vi "BooleanCtlTest.vi"() -> ()   [LabVIEW 2016]
uses:
  main/apis/Setup/GetVI/GetVIByPath.vi
  main/apis/Stimulus/ValueSignal/ValueSignalByPathString.vi
  main/apis/Assert/AssertControlValue/Equal.vi
  main/Drona.lvlib
  main/apis/Setup/GetVI/GetVI.lvlib
  <vilib>/addons/_JKI Toolkits/Caraya/classes/Test/Test.lvclass
  main/apis/Stimulus/ValueSignal/ValueSignal.lvlib
  main/apis/Assert/AssertControlValue/AssertControlValue.lvlib
panel:
  out "error out":errorcluster
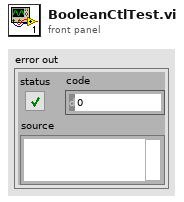
[diagram p1: front panel]
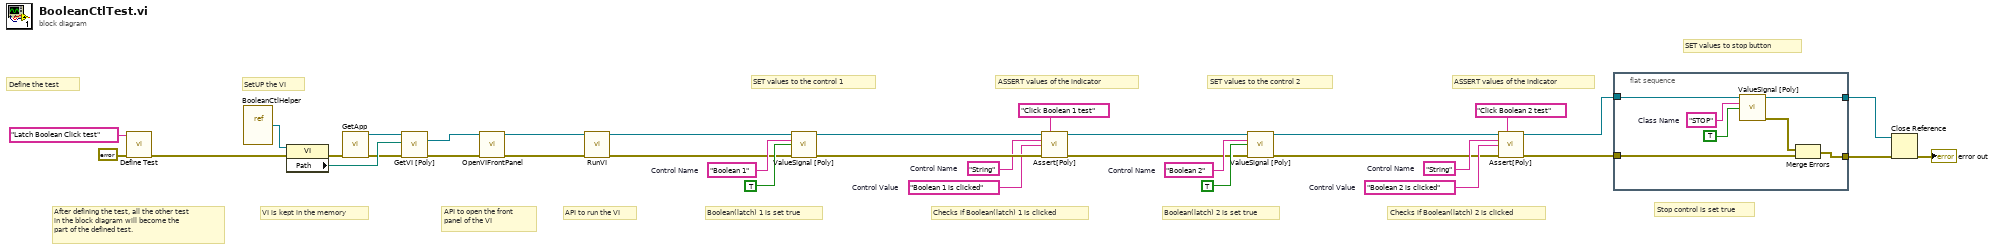
[diagram p0: block diagram]
diagram:
  w18 = "String"  # Control Name
  w14 = "Boolean 2 is clicked"  # Control Value
  w16 = "Boolean 2"  # Control Name
  w21 = "String"  # Control Name
  w26 = "Boolean 1 is clicked"  # Control Value
  w24 = "Boolean 1"  # Control Name
  # "Stop control is set true"
  # "SET values to stop button"
  # "API to open the front\npanel of the VI"
  # "Checks if Boolean(latch) 2 is clicked"
  # "ASSERT values of the indicator"
  # "Boolean(latch) 2 is set true"
  # "SET values to the control 2"
  # "Checks if Boolean(latch) 1 is clicked"
  # "ASSERT values of the indicator"
  # "Boolean(latch) 1 is set true"
  # "API to run the VI"
  # "SET values to the control 1"
  # "VI is kept in the memory"
  # "SetUP the VI"
  # "After defining the test, all the other test\nin the block diagram will become the \npart of the defined test."
  # "Define the test"
  n1 = call <vilib>:"Define Test.vi"("error in (no error)"=errorcluster {"status"=FALSE, "code"=0, "source"=""}, "Label (VI Title)"="Latch Boolean Click test") -> ("error out"=w30:errorcluster)  [unwired: 9 in]
  n2 = vi-ref "BooleanCtlHelper.vi"() -> (w23:refnum<vi>)
  n3 = property on="Property Node" class="VI"(reference=w23, error in=w30) -> (error out=w34:errorcluster, "Path"=w33:path)  [unwired: 1 out]
  n4 = call "GetApp.vi"("error in (no error)"=w34) -> ("Application Ref"=w35:refnum<vi>, "error out"=w32:errorcluster)  [unwired: 13 in]
  n5 = call-poly "GetVI [Poly].vi"("Application Ref in"=w35, "VI Path"=w33, "error in (no error)"=w32) -> ("VI Reference"=w6:refnum<vi>, "error out"=w8:errorcluster)  [unwired: 10 in, 1 out]
  n6 = call "OpenVIFrontPanel.vi"("VI Reference In"=w6, "error in"=w8) -> ("VI Reference Out"=w5:refnum<vi>, "error out"=w7:errorcluster)  [unwired: 12 in]
  n7 = call "RunVI.vi"("VI Reference In"=w5, "error in"=w7) -> ("VI Reference Out"=w20:refnum<vi>, "error out"=w19:errorcluster)  [unwired: 12 in]
  n8 = call-poly "ValueSignal [Poly].vi"("VI Reference In"=w20, "Control Path"=w24, "Value (Signaling)"=TRUE, "error in"=w19) -> ("VI Reference Out"=w27:refnum<vi>, "error out"=w28:errorcluster)  [unwired: 10 in]
  n9 = call-poly "Assert[Poly].vi"("VI Reference In"=w27, "Label"="Click Boolean 1 test" ("Label (VI Title)"), "Control Path"=w21, "Control Value"=w26, "Error In"=w28) -> ("VI Reference Out"=w10:refnum<vi>, "Error Out"=w11:errorcluster)  [unwired: 9 in]
  n10 = call-poly "ValueSignal [Poly].vi"("VI Reference In"=w10, "Control Path"=w16, "Value (Signaling)"=TRUE, "error in"=w11) -> ("VI Reference Out"=w13:refnum<vi>, "error out"=w12:errorcluster)  [unwired: 10 in]
  n11 = call-poly "Assert[Poly].vi"("VI Reference In"=w13, "Label"="Click Boolean 2 test" ("Label (VI Title)"), "Control Path"=w18, "Control Value"=w14, "Error In"=w12) -> ("VI Reference Out"=w2:refnum<vi>, "Error Out"=w4:errorcluster)  [unwired: 9 in]
  n12 = flat-sequence {
    tunnel: [w39] -> w3
    tunnel: [w40] -> w1
    tunnel: w2 -> [w38]
    tunnel: w4 -> [w36]
    frame #0 {
      w42 = "STOP"  # Class Name
      n13 = call-poly "ValueSignal [Poly].vi"("VI Reference In"=w38, "Control Path"=w42, "Value (Signaling)"=TRUE) -> ("VI Reference Out"=w40:refnum<vi>, "error out"=w37:errorcluster)  [unwired: 11 in]
      n14 = Merge Errors(w37, w36) -> (w39:errorcluster)
    }
  }
  n15 = Close Reference(reference=w1, error in (no error)=w3) -> (error out=→"error out":errorcluster)
